vi "Dashboard Main.vi"() -> ()   [LabVIEW 2015]
uses:
  <vilib>/Utility/miscctls.llb/LVRowAndColumnTypeDef.ctl
  <vilib>/event_ctls.llb/eventvkey.ctl
  <vilib>/Rock Robotics/Network Tables/NT Read Boolean.vi
  <vilib>/Rock Robotics/WPI/Dashboard/WPI_DashboardLogging Global.vi
  <vilib>/Rock Robotics/Network Tables/NT Read Numeric Array.vi
  <vilib>/Utility/config.llb/Write Key (String).vi
  <vilib>/Utility/config.llb/Write Key (I32).vi
  <vilib>/Utility/config.llb/NI_LVConfig.lvlib
  <vilib>/vision/NI_Vision_Development_Module.lvlib
panel:
  out "Camera Image 2":T1(plugin-control)
  in  "Vision 2":u16(ring) items=["Camera Off", "USB Camera SW", "USB Camera HW", "IP Camera"]
  in  "Rec Mode":enum32{"Stop", "Record", "Playback"}(radio)
  in  "Vision":u16(ring) items=["Camera Off", "USB Camera SW", "USB Camera HW", "IP Camera"]
  in  "Dashboard Tab":T2(tab)
  out "Camera Reversed":bool
  out "dist":dbl
  in  "Select Auto":string(combo)
  out "NT Connection":bool
  in  "Camera Settings":T3={"Frame Rate"=30, "Compression"=30, "Size"=1} {"Frame Rate" scale=1.0..30.0; "Size" items=["640x480", "320x240", "160x120"]}
  out "MotorChart R":cluster{"Numeric":dbl, "Numeric":dbl}(graph)
  out "MotorChart L":T4(graph)
  out "MotorSliders R":cluster{"MotorSlide1":dbl, "MotorSlide2":dbl} {"MotorSlide2" scale=-1.0..1.0 scale format="%#_2e"; "MotorSlide1" scale=-1.0..1.0 scale format="%#_2e"}
  out "MotorSliders L":T5 {"MotorSlide4 2" scale=0.0..14.0 scale format="%#_2e"; "MotorSlide2" scale=-1.0..1.0 scale format="%#_2e"; "MotorSlide1" scale=-1.0..1.0 scale format="%#_2e"}
  out "Gyro":dbl(knob) scale=0.0..360.0
  out "JS1 Z":dbl(slide) scale=-1.0..1.0 scale format="%#_2e"
  out "JS1 Graph":cluster{"X":dbl, "Y":dbl}[](graph)
  out "JS1 Buttons":T6
  out "JS2 Z":dbl(slide) scale=-1.0..1.0 scale format="%#_2e"
  out "JS2 Graph":cluster{"X":dbl, "Y":dbl}[](graph)
  out "JS2 Buttons":T6
  out "Mode":T7(ring)=enum."Auto Disabled"
  in  "DB Camera Config":bool
  out "fps":dbl format="%#.1g"
  out "Mbps":dbl format="%#.1g"
  out "Mbps LED":bool
  in  "Camera Settings 2":T3={"Frame Rate"=30, "Compression"=30, "Size"=1} {"Frame Rate" scale=1.0..30.0; "Size" items=["640x480", "320x240", "160x120"]}
  out "Mbps 2":dbl format="%#.1g"
  out "fps 2":dbl format="%#.1g"
  out "Background":bool
  in  "DB/String 9":string
  in  "DB/String 8":string
  in  "DB/String 7":string
  in  "DB/String 6":string
  in  "DB/String 5":string
  in  "DB/String 4":string
  in  "DB/String 3":string
  in  "DB/String 2":string
  in  "DB/String 1":string
  in  "DB/String 0":string
  in  "DB/Slider 0":dbl(slide) scale=0.0..5.0
  in  "DB/Slider 1":dbl(slide) scale=0.0..5.0
  in  "DB/Slider 2":dbl(slide) scale=0.0..5.0
  in  "DB/Slider 3":dbl(slide) scale=0.0..5.0
  out "DB/LED 3":bool
  out "DB/LED 2":bool
  out "DB/LED 1":bool
  out "DB/LED 0":bool
  in  "DB/Button 3":bool
  in  "DB/Button 2":bool
  in  "DB/Button 1":bool
  in  "DB/Button 0":bool caption="New Name"
  in  "Test Slider":dbl(slide) scale=0.0..100.0 scale format="%#_3g"
  in  "On/Off":bool caption="Solenoid"
  in  "Test Name":u16(ring) items=["Select the test to run..."]
  in  "Test Tree":string(tree)
  in  "Motor":cluster{"Value":dbl, "Enable":bool} {"Value" scale=-1.0..1.0 scale format="%#_3g"}
  out "Progress":T8 {"Test Progress" scale=0.0..100.0}
  in  "Rev/Fwd":cluster{"Forward":bool, "Reverse":bool}
  in  "Test Ring":u16(ring) items=["Monochrome", "Color"]
  out "Cmd Status":string
  in  "Execute Command":bool
  in  "Command Params":string[][](table)
  in  "Command Selection":i32(listbox)
  in  "CheckList":i32(listbox)
  out "Tree":string(tree)
  in  "TCP":refnum<k5>
  out "Camera IP":string
  out "Image Message":string="Timeout in Camera Communications"
  out "Camera Image":T1(plugin-control)
  # "Left"
  # "Front"
  # "Right"
  # "Battery"
  # "This tab is a great place for autonomous settings and robot-specific values.\nPlace controls and indicators inside this tab and match name to\nDashboard Variables on robot. You can also delete this comment."
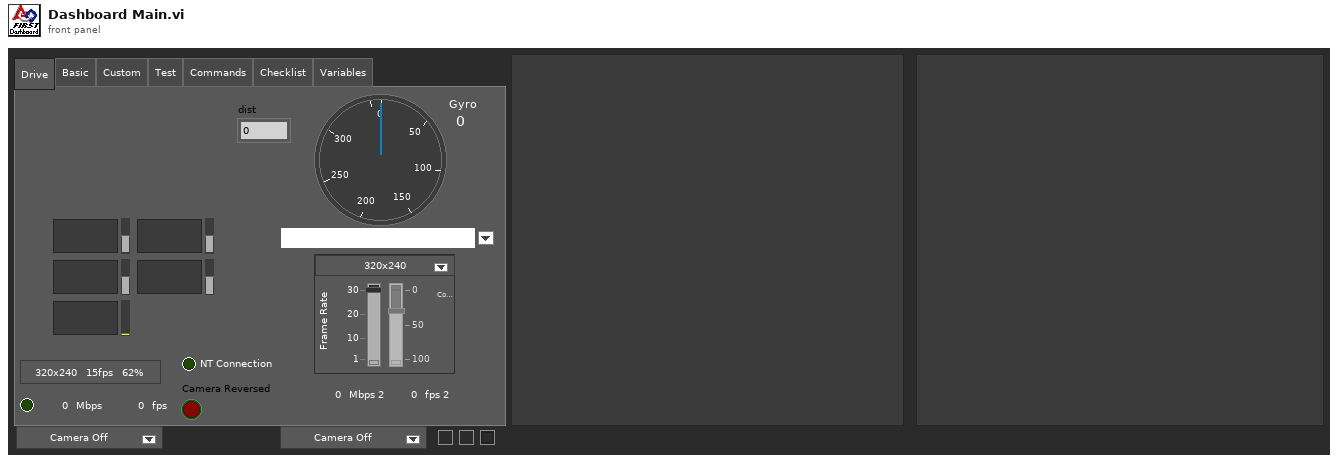
[diagram p1: front panel]
types:
  T1 = typedef "IMAQ Image.ctl" = refnum<image>
  T2 = enum32{"Drive", "Basic", "Custom", "Test", "Commands", "Checklist", "Variables"}
  T3 = cluster{"Frame Rate":i32, "Compression":i32, "Size":u16}
  T4 = cluster{"Numeric":dbl, "Numeric":dbl, "Battery V":dbl}
  T5 = cluster{"MotorSlide1":dbl, "MotorSlide2":dbl, "MotorSlide4 2":dbl}
  T6 = cluster{bool, bool, bool, bool, bool, bool, bool, bool, bool, bool, bool, bool}
  T7 = enum8{"Tele-Op Disabled", "Tele-Op Enabled", "Auto Disabled", "Auto Enabled", "Test Disabled", "Test Enabled", "Disconnected", "No Code", "E-Stop"}
  T8 = cluster{"Test Progress":u8, "Test Progress Text":string}
  T9 = cluster{"IDs":cluster{"RPC field ID":u16, "Unique ID":u16}, "String":string}
  T10 = enum32{"Drive", "Basic", "Custom", "Test", "Checklist", "Variables"}
  T11 = typedef "Image Type" = u32
  T12 = cluster{"Camera Image":refnum<vi>, "Dashboard Tab":refnum<vi>, "Background":refnum<vi>, "Vision":refnum<vi>, "Rec Mode":refnum<vi>, "Test Slider":refnum<vi>, "On/Off ":refnum<vi>, "Test Ring":refnum<vi>, "Rev/Fwd":refnum<vi>, "Test Name":refnum<vi>, "Motor":refnum<vi>, "Progress":refnum<vi>, "CheckList":refnum<vi>, "Tree":refnum<vi>, "Test Tree":refnum<vi>, "Command Params":refnum<vi>, "Command Selection":refnum<vi>, "Execute Command":refnum<vi>, "Cmd Status":refnum<vi>}
  T13 = cluster{"Error Strings":string, "Disable Counts":cluster{u16, u16}, "Rail Faults":cluster{u16, u16, u16}, "Robot IP":string, "DB Mode":u8, "Event Info":cluster{"Name":string, "Type":u8, "Number":u16, "Replay":u8}, "Camera Addr":string}
  T14 = cluster{"Storage":cluster{"Disk Free":u64, "RAM Block":u32, "RAM free":u32}, "CPU Utilization":cluster{"CPU % ISR":sgl, "CPU % Time Crit":sgl, "CPU % Timed Str":sgl, "CPU % High":sgl, "CPU % Above":sgl, "CPU % Normal":sgl, "CPU % Low":sgl}, "CAN":cluster{"% Bus Utilization":sgl, "Bus Off Cnt":u32, "TX_FIFO Full Cnt":u32, "Receive Error Cnt":u8, "Transmit Error Cnt":u8}, "HID":cluster{"HID Outputs":u32, "Rumble Low":u16, "Rumble High":u16}[]}
  T15 = cluster{"Status bits":cluster{"Test Mode":bool, "Autonomous":bool, "Enabled":bool, "Code Start":bool, "Brownout":bool, "Reserved 2":bool, "Reserved 3":bool, "E-Stop":bool}, "Code Trace":cluster{"Disabled":bool, "TeleOp":bool, "Auto":bool, "Test":bool}, "Controller Type":enum16{"unknown", "cRIO", "roboRio"}, "Code?":enum16{"unknown", "noCode", "code"}, "Battery V":dbl}
  T16 = cluster{"Control Bits":cluster{"TestMode":bool, "Autonomous":bool, "Enabled":bool, "FMS Present":bool, bool, bool, bool, "E-Stop":bool}, "Team Station ":u8, "Countdown":sgl, "Joystick Values":cluster{"Axes":dbl[], "Buttons":bool[], "POVs":i16[]}[]}
  T17 = cluster{"Axes":dbl[], "Buttons":bool[], "POVs":i16[]}[]
  T18 = cluster{"Axes":dbl[], "Buttons":bool[], "POVs":i16[]}
  T19 = cluster{"Buttons[0]":bool, "Buttons[1]":bool, "Buttons[2]":bool, "Buttons[3]":bool, "Buttons[4]":bool, "Buttons[5]":bool, "Buttons[6]":bool, "Buttons[7]":bool, "Buttons[8]":bool, "Buttons[9]":bool, "Buttons[10]":bool, "Buttons[11]":bool}
  T20 = typedef "NI_LVConfig.lvlib/Config Data RefNum.ctl" = refnum<k1>
  T21 = cluster{"Operation":enum16{"Update", "Clear"}, "Color Box":u32}[]
  T22 = typedef "eventvkey.ctl" = enum16{"ASCII", "Enter", "Return", "Shift", "Ctrl", "Alt", "Cmd", "Opt", "Caps", "NumLock", "Clear", "Break", "Up", "Down", "Left", "Right", "Insert", "Delete", "Home", "End", "PageUp", "PageDown", "Escape", "Help", "Pause", "ScrollLock", "F1", "F2", "F3", "F4", "F5", "F6", "F7", "F8", "F9", "F10", "F11", "F12", "F13", "F14", "F15", "F16", "F17", "F18", "F19", "F20", "F21", "F22", "F23", "F24", "Play", "VolumeUp", "VolumeDown", "Mute", "Two Byte Char"}
  T23 = cluster{"Image Size":bool, "Image Type":bool, "Pixel Value":bool, "ROI Information":bool, "Zoom Factor":bool}
  T24 = enum8{"Enabled", "Disabled", "Disabled and Grayed Out"}
  T25 = cluster{"Operation":enum16{"Update", "Clear"}, "Color Box":u32}
  T26 = typedef "LVRowAndColumnTypeDef.ctl" = cluster{"Row":i32, "Column":i32}
  T27 = cluster{"Shift":bool, "Ctrl":bool, "Alt":bool, "Cmd":bool, "Opt":bool}
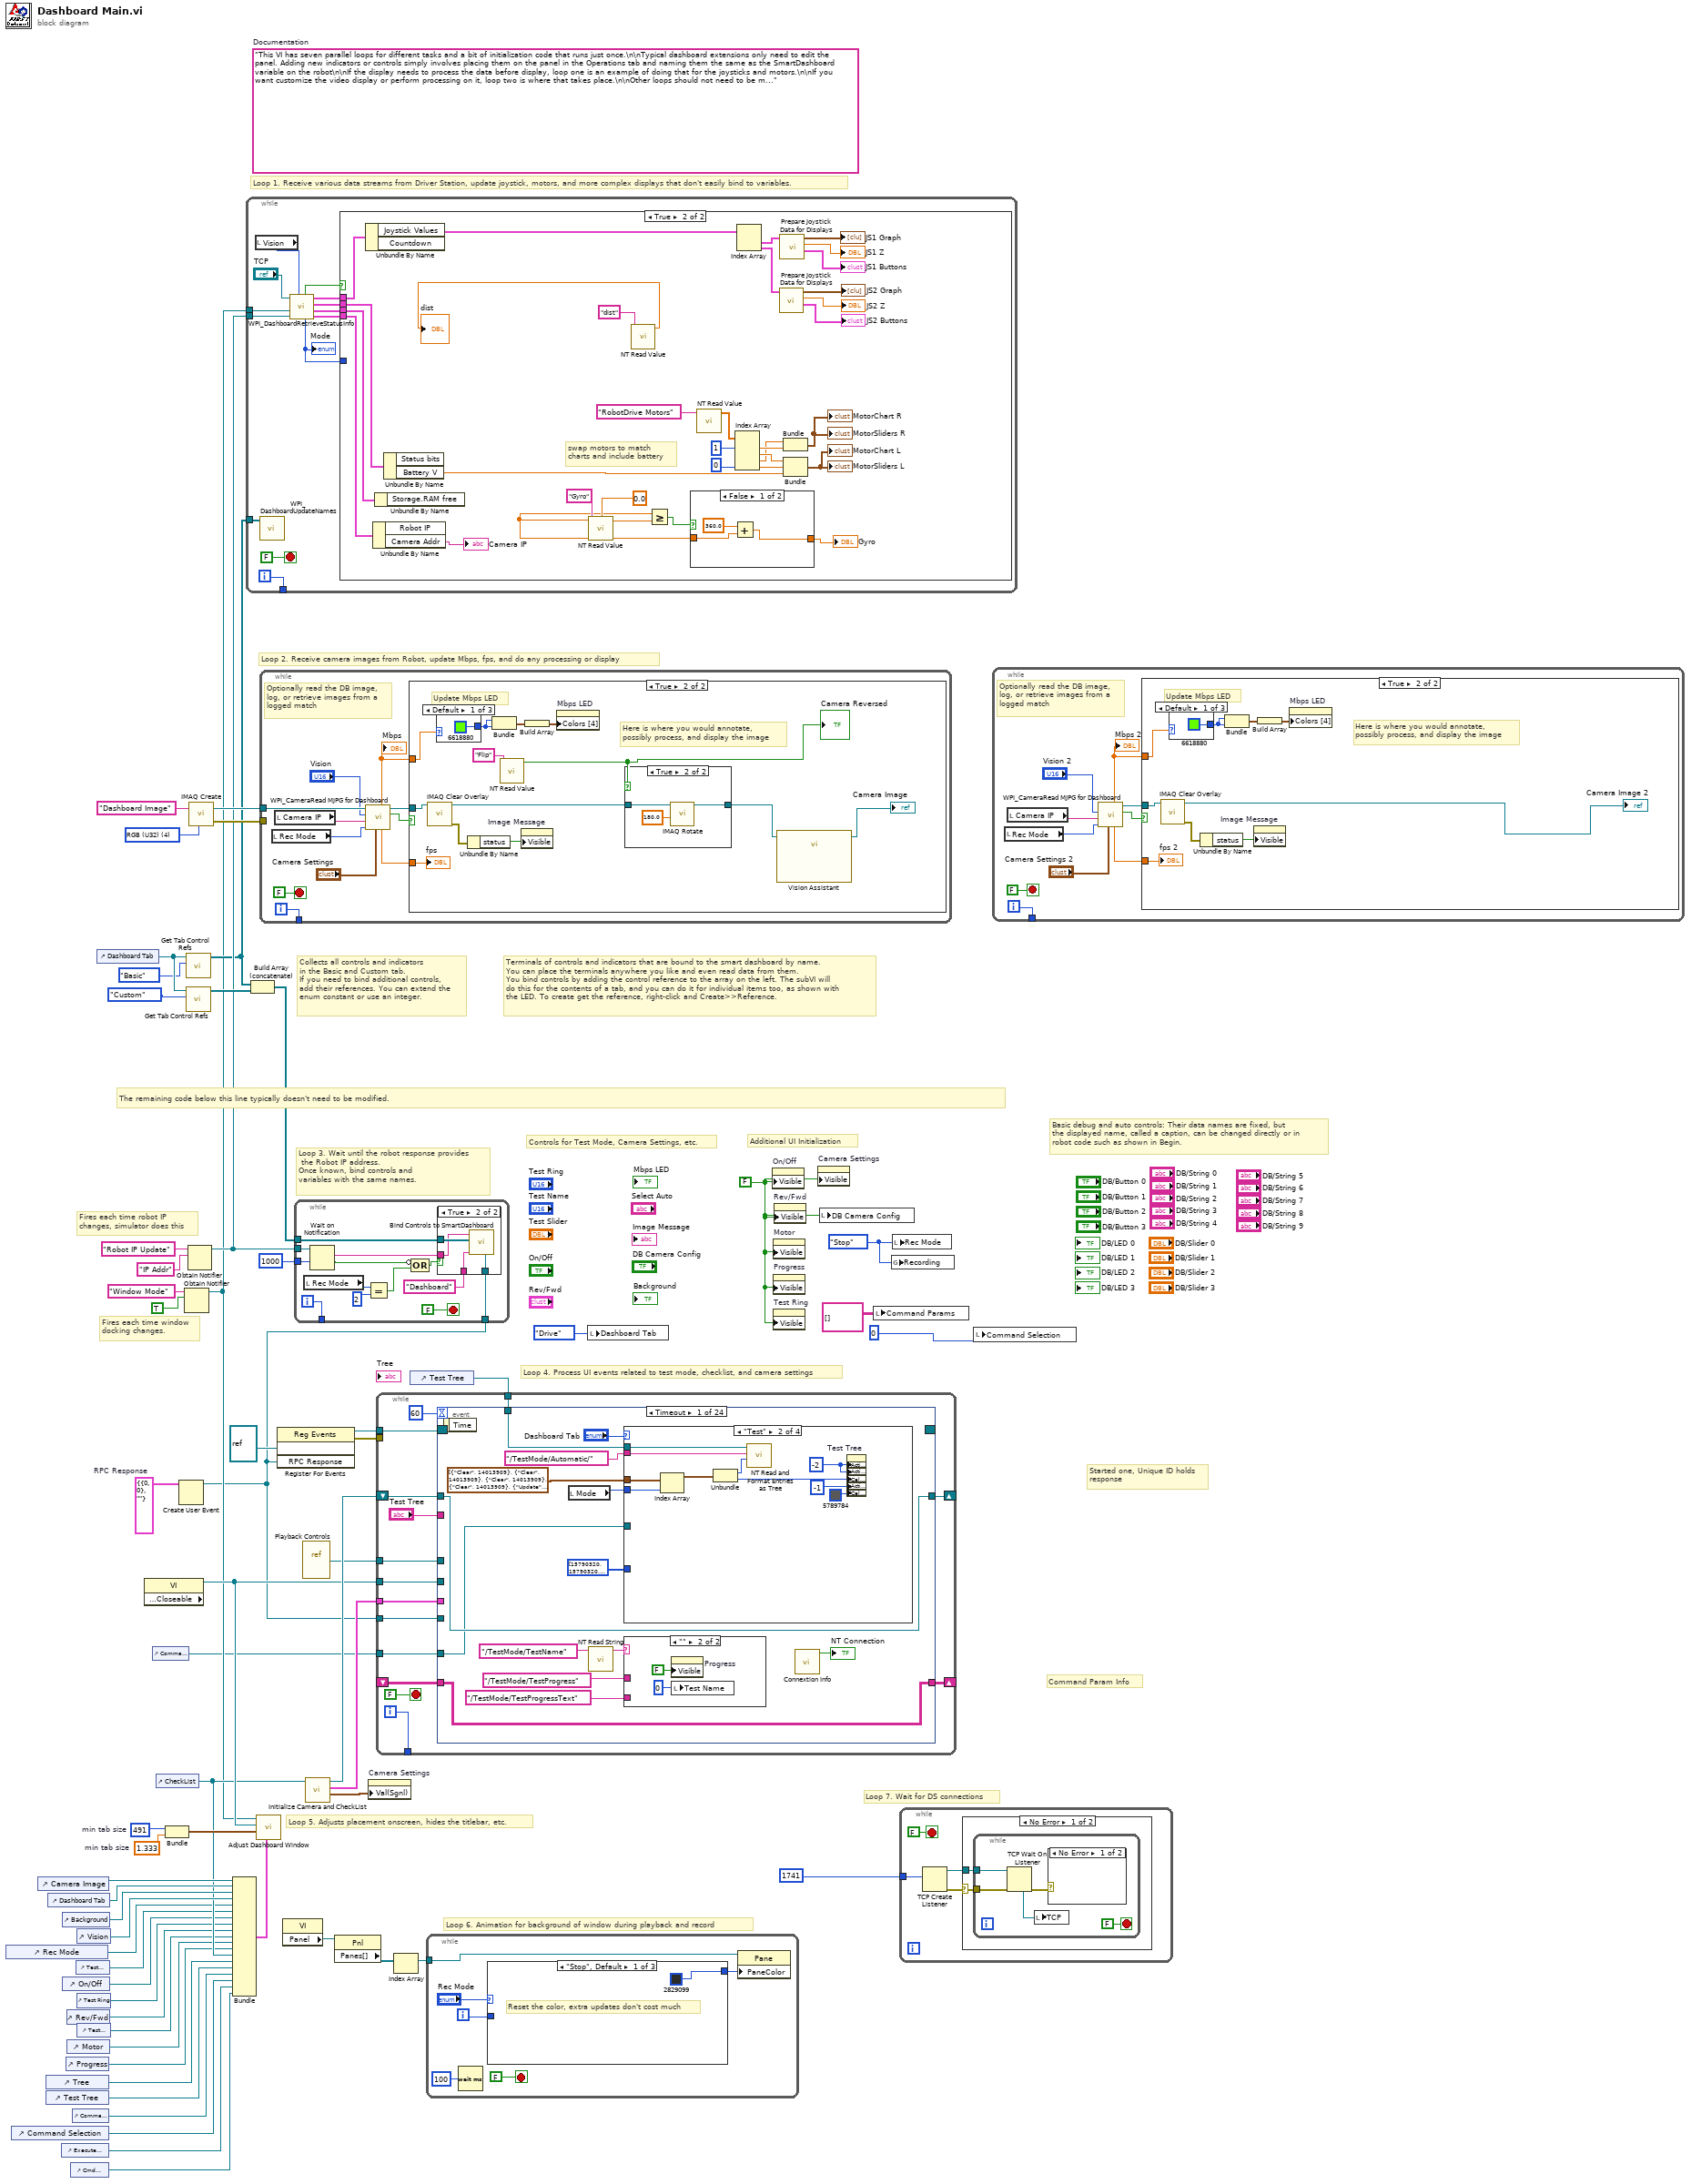
[diagram p0: block diagram]
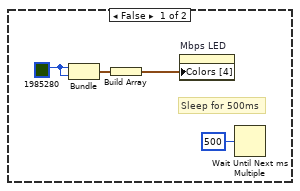
[diagram p2: hidden frame]
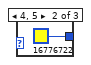
[diagram p3: hidden frame]
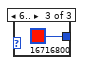
[diagram p4: hidden frame]
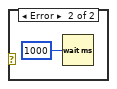
[diagram p5: hidden frame]
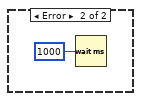
[diagram p6: hidden frame]
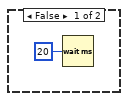
[diagram p7: hidden frame]
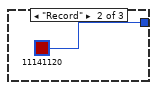
[diagram p9: hidden frame]
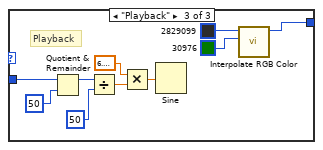
[diagram p10: hidden frame]
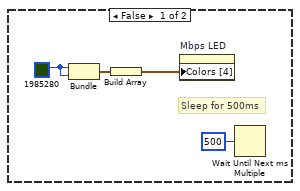
[diagram p12: hidden frame]
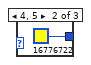
[diagram p14: hidden frame]
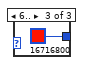
[diagram p15: hidden frame]
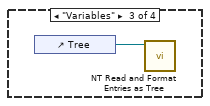
[diagram p17: hidden frame]
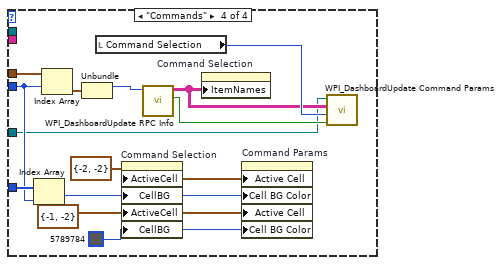
[diagram p18: hidden frame]
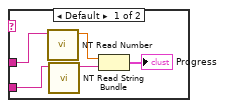
[diagram p19: hidden frame]
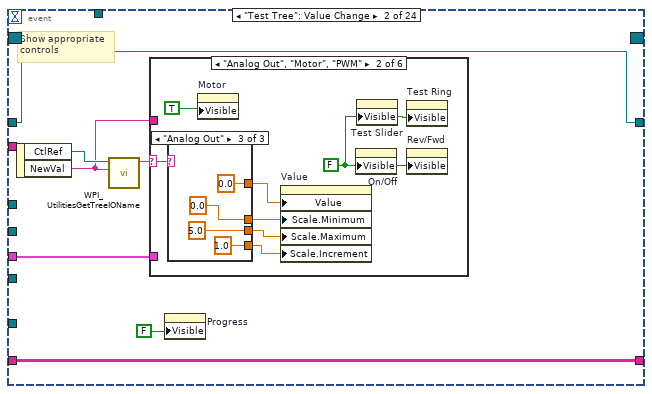
[diagram p20: hidden frame]
diagram:
  w7 = T9 {"IDs"={"RPC field ID"=0, "Unique ID"=0}, "String"=""}  # RPC Response
  w33 = 491  # min tab size
  w32 = 1.333  # min tab size
  w41 = enum32{"Stop", "Record", "Playback"}."Stop" ("Rec Mode")
  w15 = FALSE ("Visible")
  (unwired) "This VI has seven parallel loops for different tasks and a bit of initialization code that runs just once.\n\nTypical dashboard extensions only need to edit the panel. Adding new indicators or controls simply involves placing them on the panel in the Operations tab and naming them the same as the SmartDashboard variable on the robot\n\nIf the display needs to process the data before display, loop one is an example of doing that for the joysticks and motors.\n\nIf you want customize the video display or perform processing on it, loop two is where that takes place.\n\nOther loops should not need to be modified. They are pretty standard, and document the task they perform."  # Documentation
  w61 = T11 4 items=["Grayscale (U8)", "Grayscale (I16)", "Grayscale (SGL)", "Complex (CSG)", "RGB (U32)", "HSL (U32)", "RGB (U64)"] ("Image Type")
  # "Command Param Info"
  # "Started one, Unique ID holds\nresponse"
  # "Loop 7. Wait for DS connections"
  # "Basic debug and auto controls: Their data names are fixed, but\nthe displayed name, called a caption, can be changed directly or in\nrobot code such as shown in Begin."
  # "Controls for Test Mode, Camera Settings, etc."
  # "Additional UI Initialization"
  # "Loop 6. Animation for background of window during playback and record"
  # "Fires each time robot IP\nchanges, simulator does this"
  # "Fires each time window\ndocking changes."
  # "Collects all controls and indicators\nin the Basic and Custom tab.\nIf you need to bind additional controls,\nadd their references. You can extend the\nenum constant or use an integer."
  # "The remaining code below this line typically doesn't need to be modified."
  # "Loop 4. Process UI events related to test mode, checklist, and camera settings"
  # "Terminals of controls and indicators that are bound to the smart dashboard by name.\nYou can place the terminals anywhere you like and even read data from them.\nYou bind controls by adding the control reference to the array on the left. The subVI will\ndo this for the contents of a tab, and you can do it for individual items too, as shown with\nthe LED. To create get the reference, right-click and Create>>Reference."
  # "Loop 3. Wait until the robot response provides\n the Robot IP address.\nOnce known, bind controls and\nvariables with the same names."
  # "Loop 5. Adjusts placement onscreen, hides the titlebar, etc."
  # "Loop 1. Receive various data streams from Driver Station, update joystick, motors, and more complex displays that don't easily bind to variables."
  # "Loop 2. Receive camera images from Robot, update Mbps, fps, and do any processing or display"
  n1 = control-ref of="Rec Mode"() -> (w21:refnum<vi>)
  n2 = control-ref of="Command Selection"() -> (w6:refnum<vi>)
  n3 = control-ref of="Camera Image"() -> (w36:refnum<vi>)
  n4 = control-ref of="Tree"() -> (w25:refnum<vi>)
  n5 = control-ref of="Test Tree"() -> (w24:refnum<vi>)
  n6 = control-ref of="Dashboard Tab"() -> (w35:refnum<vi>)
  n7 = control-ref of="Execute Command"() -> (w8:refnum<vi>)
  n8 = control-ref of="Background"() -> (w30:refnum<vi>)
  n9 = control-ref of="On/Off"() -> (w19:refnum<vi>)
  n10 = control-ref of="Progress"() -> (w16:refnum<vi>)
  n11 = control-ref of="Rev/Fwd"() -> (w17:refnum<vi>)
  n12 = control-ref of="Motor"() -> (w22:refnum<vi>)
  n13 = control-ref of="Cmd Status"() -> (w2:refnum<vi>)
  n14 = control-ref of="Command Params"() -> (w9:refnum<vi>)
  n15 = control-ref of="Test Slider"() -> (w20:refnum<vi>)
  n16 = control-ref of="Vision"() -> (w34:refnum<vi>)
  n17 = control-ref of="Test Ring"() -> (w18:refnum<vi>)
  n18 = control-ref of="Test Name"() -> (w23:refnum<vi>)
  n19 = control-ref of="Dashboard Tab"() -> (w39:refnum<vi>)
  n20 = property class="VI" props=["Front Panel.Closeable"]() -> (reference out=w40:refnum<vi>)  [unwired: 2 in, 2 out]
  n21 = control-ref of="Command Params"() -> (w1:refnum<vi>)
  n22 = control-ref of="CheckList"() -> (w26:refnum<vi>)
  n23 = Bundle("min tab size"=w33, "min tab size"=w32) -> (w31:cluster{"min tab size":i32, "min tab size":dbl})  [unwired: 1 in]
  n24 = Create User Event(user event datatype=w7) -> (user event=w3:refnum<user-event>)  [unwired: 1 in, 1 out]
  n25 = Obtain Notifier(name (unnamed)="Window Mode", notification data type=TRUE) -> (notifier out=w12:refnum<notifier>)  [unwired: 2 in, 2 out]
  n26 = call <vilib>:"Get Tab Control Refs.vi"("Page Index"=T10."Basic" ("Dashboard Tab"), "TabControl in"=w39) -> ("ControlsOnPage"=w13:refnum<vi>[])  [unwired: 9 in]
  n27 = call <vilib>:"Get Tab Control Refs.vi"("Page Index"=T10."Custom" ("Dashboard Tab"), "TabControl in"=w39) -> ("ControlsOnPage"=w38:refnum<vi>[])  [unwired: 9 in]
  n28 = Obtain Notifier(name (unnamed)="Robot IP Update", notification data type="IP Addr" ("name (unnamed)")) -> (notifier out=w14:refnum<notifier>)  [unwired: 2 in, 2 out]
  n29 = call "IMAQ Create"("Image Name"="Dashboard Image", "Image Type"=w61) -> ("New Image"=w59:T1, "error out"=w58:errorcluster)  [unwired: 2 in, 1 out]
  n30 = Bundle("Camera Image"=w36, "Dashboard Tab"=w35, "Background"=w30, "Vision"=w34, "Rec Mode"=w21, "Test Slider"=w20, "On/Off"=w19, "Test Ring"=w18, "Rev/Fwd"=w17, "Test Name"=w23, "Motor"=w22, "Progress"=w16, "CheckList"=w26, "Tree"=w25, "Test Tree"=w24, "Command Params"=w9, "Command Selection"=w6, "Execute Command"=w8, "Cmd Status"=w2) -> (w27:T12)  [unwired: 1 in]
  n31 = while {
    tunnel: [w73] -> _
    tunnel: w14 -> [w67]
    tunnel: w13 -> [w66]
    tunnel: w12 -> [w62]
    i -> [w73]
    stop <- FALSE stop-if-true
    n32 = local read "Vision"() -> (w64:u16)
    n33 = call <vilib>:"WPI_DashboardUpdateNames.vi"("Controls on Tab"=w66) -> ()  [unwired: 11 in]
    n34 = call <vilib>:"WPI_DashboardRetrieveStatusInfo.vi"("Vision"=w64, "Binding Refnum"=w67, "Window Mode Notifier"=w62, "TCP Cnx"="TCP") -> ("Power and Errors"=w68:T13, "Robot Metrics"=w71:T14, "Status Info"=w72:T15, "Control Info"=w69:T16, "Robot Mode"=w65:T7, "Process?"=w70:bool)  [unwired: 2 in]
    "Mode" <- w65
    n35 = case shown="True" w70 {
      tunnel: w72 -> [_ w107]
      tunnel: w71 -> [_ w106]
      tunnel: w69 -> [_ w105]
      tunnel: w68 -> [_ w104]
      tunnel: w65 -> [_ _]
      frame False {
        n36 = Wait (ms)(milliseconds to wait=u32 20) -> ()  [unwired: 1 out]
      }
      frame True {
        # "swap motors to match\ncharts and include battery"
        n37 = Unbundle By Name(w105) -> ("Joystick Values"=w94:T17)  [unwired: 1 out]
        n38 = Unbundle By Name(w104) -> ("Camera Addr"=→"Camera IP":string)  [unwired: 1 out]
        n39 = Unbundle By Name(w106) -> ()  [unwired: 1 out]
        n40 = Unbundle By Name(w107) -> ("Battery V"=w95:dbl)  [unwired: 1 out]
        n41 = call-poly <vilib>:"NT Read Value.vi"("Name"="Gyro") -> ("Numeric"=w79:dbl)  [unwired: 9 in, 1 out]
        n42 = call-poly <vilib>:"NT Read Value.vi"("Name"="dist") -> ("Numeric"=→"dist":dbl)  [unwired: 9 in, 1 out]
        n43 = Greater Or Equal?(x=w79, y=0.0) -> (x >= y?=w81:bool)
        n44 = case shown="False" w81 {
          tunnel: [w108 w111] -> w78
          tunnel: w79 -> [w109 w111]
          frame False {
            n45 = Add(x=360.0, y=w109) -> (x+y=w108:dbl)
          }
          frame True {
          }
        }
        "Gyro" <- w78
        n46 = call-poly <vilib>:"NT Read Value.vi"("Name"="RobotDrive Motors") -> ("Numeric Array"=w83:dbl[])  [unwired: 9 in, 1 out]
        n47 = Index Array(array=w83, index #1=1, index #4=0) -> (element #1=w99:dbl, element #2=w100:dbl, element #3=w98:dbl, element #4=w103:dbl)  [unwired: 2 in]
        n48 = Index Array(array=w94) -> (element #1=w93:T18, element #2=w88:T18)  [unwired: 2 in]
        n49 = call "Prepare Joystick Data for Displays.vi"("Joystick Values"=w88) -> ("Buttons"=→"JS2 Buttons":T19, "Z Axis"=→"JS2 Z":dbl, "Cartesian Data"=→"JS2 Graph":cluster{"X axis":dbl, "X axis":dbl}[])  [unwired: 8 in]
        n50 = call "Prepare Joystick Data for Displays.vi"("Joystick Values"=w93) -> ("Buttons"=→"JS1 Buttons":T19, "Z Axis"=→"JS1 Z":dbl, "Cartesian Data"=→"JS1 Graph":cluster{"X axis":dbl, "X axis":dbl}[])  [unwired: 8 in]
        n51 = Bundle("Numeric"=w98, "Numeric"=w99) -> (→"MotorChart R" →"MotorSliders R":cluster{"Numeric":dbl, "Numeric":dbl})  [unwired: 1 in]
        n52 = Bundle("Numeric"=w100, "Numeric"=w103, "Battery V"=w95) -> (→"MotorChart L" →"MotorSliders L":T4)  [unwired: 1 in]
      }
    }
  }
  n53 = Build Array (concatenate)(w13, w38) -> (w37:refnum<vi>[])
  n54 = call "Adjust Dashboard Window.vi"("Sizing Refnums"=w27, "Size Constraints"=w31, "VI"=w40, "WIn Mode"=w12) -> ()  [unwired: 8 in]
  n55 = while {
    tunnel: w59 -> [w120]
    tunnel: w58 -> [_]
    tunnel: [w121] -> _
    i -> [w121]
    stop <- FALSE stop-if-true
    # "Optionally read the DB image,\nlog, or retrieve images from a\nlogged match"
    n56 = local read "Rec Mode"() -> (w115:enum32{"Stop", "Record", "Playback"})
    n57 = local read "Camera IP"() -> (w113:string)
    n58 = call <vilib>:"WPI_CameraRead MJPG for Dashboard.vi"("Camera Settings"="Camera Settings", "Rec Mode"=w115, "Camera IP"=w113, "Camera Mode"="Vision", "Refnum in"=w120) -> ("Active"=w118:bool, "Refnum out"=w119:T1, "FPS"=w117:dbl, "Bandwidth (Mbps)"=w112:dbl)  [unwired: 3 in]
    "Mbps" <- w112
    n59 = case shown="True" w118 {
      tunnel: w119 -> [_ w134]
      tunnel: w112 -> [_ w133]
      tunnel: w117 -> [_ w132]
      frame False {
        w123 = u32 1985280 ("Color Box")
        # "Sleep for 500ms"
        n60 = Bundle("Color Box"=w123, "Color Box"=w123) -> (w125:cluster{"Color Box":u32, "Color Box":u32})  [unwired: 1 out]
        n61 = Build Array(w125) -> (w124:cluster{"Color Box":u32, "Color Box":u32}[])
        n62 = property on="Mbps LED" class="Bool (strict)"("Colors [4]"=w124) -> ()  [unwired: 2 in, 2 out]
        n63 = Wait Until Next ms Multiple(millisecond multiple=u32 500) -> ()  [unwired: 1 out]
      }
      frame True {
        # "Here is where you would annotate,\npossibly process, and display the image"
        # "Update Mbps LED"
        n64 = call "IMAQ Clear Overlay"("Image"=w134) -> ("error out"=w138:errorcluster, "Image Out"=w131:T1)  [unwired: 2 in, 7 out]
        n65 = case shown="Default" w133 {
          tunnel: [u32 6618880 ("Color Box") u32 16776722 ("Color Box") u32 16716800 ("Color Box")] -> w135
          frame Default {
          }
          frame 4, 5 {
          }
          frame 6.. {
          }
        }
        n66 = Unbundle By Name(w138) -> ("status"=w139:bool)
        n67 = Bundle("Color Box"=w135, "Color Box"=w135) -> (w137:cluster{"Color Box":u32, "Color Box":u32})  [unwired: 1 out]
        n68 = call-poly <vilib>:"NT Read Value.vi"("Name"="Flip") -> ("Boolean"=w129:bool)  [unwired: 9 in, 1 out]
        "Camera Reversed" <- w129
        n69 = property on="Image Message" class="Str"("Visible"=w139) -> ()  [unwired: 2 in, 2 out]
        n70 = Build Array(w137) -> (w136:cluster{"Color Box":u32, "Color Box":u32}[])
        n71 = property on="Mbps LED" class="Bool (strict)"("Colors [4]"=w136) -> ()  [unwired: 2 in, 2 out]
        n72 = case shown="True" w129 {
          tunnel: w131 -> [w140 w143]
          tunnel: [w140 w142] -> w128
          frame False {
          }
          frame True {
            n73 = call "IMAQ Rotate"("Angle (degrees)"=sgl 180.0, "Image Src"=w143) -> ("Image Dst Out"=w142:T1)  [unwired: 8 in, 1 out]
          }
        }
        n74 = call "Vision Assistant"("Image In"=w128) -> ("Image Out"=→"Camera Image":T1)  [unwired: 25 in, 1 out]
        "fps" <- w132
      }
    }
  }
  n75 = register-events(refnum<vi> refnum, w3) -> (reference out=w45:refnum<event-registration>, error out=w44:errorcluster)  [unwired: 2 in]
  n76 = property class="VI"() -> ("Panel"=w48:refnum<vi>)  [unwired: 2 in, 2 out]
  n77 = while {
    tunnel: w37 -> [w159]
    tunnel: w14 -> [w157]
    tunnel: [w155] -> _
    tunnel: u32 1000 ("milliseconds to wait") -> [w154]
    tunnel: w3 -> [w147]
    i -> [w155]
    stop <- FALSE stop-if-true
    n78 = local read "Rec Mode"() -> (w150:enum32{"Stop", "Record", "Playback"})
    n79 = Wait on Notification(notifier=w157, timeout in ms (-1)=w154) -> (notification=w156:string, timed out?=w152:bool)  [unwired: 2 in, 2 out]
    n80 = Equal?(x=w150, y=u16 2 ("Rec Mode")) -> (x = y?=w151:bool)
    n81 = Compound Arithmetic op=OR(invert w152, w151) -> (w153:bool)
    n82 = case shown="True" w153 {
      tunnel: w159 -> [_ w163]
      tunnel: w156 -> [_ w162]
      tunnel: "Dashboard" -> [_ w161]
      tunnel: w147 -> [_ w160]
      frame False {
      }
      frame True {
        n83 = call <vilib>:"Bind Controls to SmartDashboard.vi"("RPC ref"=w160, "Client Name"=w161, "Bound Control Refs"=w163, "Server IP Address"=w162) -> ()  [unwired: 8 in]
      }
    }
  }
  n84 = vi-ref "Playback Controls.vi"() -> (w46:refnum<vi>)
  n85 = call "Initialize Camera and CheckList.vi"("ListBox in"=w26) -> ("Cluster"=w52:cluster{"value":i32, "value":i32, "index":i32}, "Array"=w53:cluster{string[]}[], "File Refnum"=w51:T20)  [unwired: 8 in]
  n86 = property class="Pnl"(reference=w48) -> ("Panes[]"=w49:refnum<vi>[])  [unwired: 1 in, 2 out]
  n87 = property on="Camera Settings" class="Clust (strict)"("Val(Sgnl)"=w52) -> ()  [unwired: 2 in, 2 out]
  n88 = Index Array(array=w49) -> (element=w47:refnum<vi>)  [unwired: 1 in]
  n89 = control-ref of="Test Tree"() -> (w50:refnum<vi>)
  n90 = while {
    tunnel: w53 -> [w175]
    shift-right: [w174] -> _
    shift-left: w51 -> [w173]
    tunnel: [w172] -> _
    tunnel: w50 -> [w171]
    tunnel: w46 -> [w170]
    tunnel: w45 -> [w169]
    tunnel: w44 -> [_]
    tunnel: w40 -> [w168]
    tunnel: w3 -> [w167]
    tunnel: w1 -> [w166]
    shift-right: [w165] -> _
    shift-left: _ -> [w164]
    i -> [w172]
    stop <- FALSE stop-if-true
    n91 = event shown="[0] Timeout" {
      selector: w169 -> [_ _ _ _ _ _ _ _ _ _ _ _ _ _ _ _ _ _ _ _ _ _ _ _]
      dyn-events: [_ _ _ _ _ _ _ _ _ _ _ _ _ _ _ _ _ _ w484 _ _ _ _ _] -> _
      timeout: u32 60 ("milliseconds to wait") -> [_ _ _ _ _ _ _ _ _ _ _ _ _ _ _ _ _ _ _ _ _ _ _ _]
      tunnel: w171 -> [w188 _ _ _ _ _ _ _ _ _ _ _ _ _ _ _ _ _ _ _ _ _ _ _]
      tunnel: "Test Tree" -> [_ _ _ _ _ _ _ _ _ _ _ _ _ w447 w456 w459 w464 w473 _ _ _ _ _ _]
      tunnel: w175 -> [_ w226 _ _ _ _ _ _ _ _ _ w409 w440 _ _ _ _ _ _ _ _ _ _ _]
      tunnel: [w185 w225 w329 w335 w345 w349 w355 w367 w375 w381 w394 w408 w433 w446 w454 w458 w463 w472 w486 w502 w504 w512 w523 w528] -> w174
      tunnel: w173 -> [w185 w225 w329 w335 w345 w349 w355 w367 w375 w381 w394 w407 w433 w446 w454 w458 w463 w472 w486 w502 w504 w512 w523 w528]
      tunnel: w170 -> [_ _ _ _ _ _ _ _ _ _ _ _ _ _ _ _ _ _ w487 _ w507 _ _ _]
      tunnel: w168 -> [_ _ _ _ _ _ _ _ _ _ _ _ _ _ _ _ _ _ w482 _ _ _ _ _]
      tunnel: w167 -> [_ _ _ _ _ _ _ _ _ _ _ _ _ _ _ _ _ _ w478 _ _ _ _ _]
      tunnel: w166 -> [w180 _ _ _ _ _ w353 _ _ _ _ _ _ _ _ _ _ _ _ _ _ _ _ _]
      tunnel: [w179 w224 w328 w334 w344 w350 w351 w361 w372 w380 w393 w406 w432 w445 w453 w457 w462 w471 w477 w500 w503 w508 w516 w529] -> w165
      tunnel: w164 -> [w179 w224 w328 w334 w344 w350 w351 _ _ w380 w393 w406 w432 w445 w453 w457 w462 w471 w477 w500 w503 w508 w516 w529]
      event Timeout {
        n92 = event-data() -> ()  [unwired: 1 in, 1 out]
        n93 = local read "Mode"() -> (w182:T7)
        n94 = call <vilib>:"NT Read String.vi"("Name"="/TestMode/TestName") -> ("String"=w191:string)  [unwired: 9 in, 1 out]
        n95 = case shown="\"Test\"" "Dashboard Tab" {
          tunnel: w188 -> [_ w202 _ _]
          tunnel: "/TestMode/Automatic/" ("Name Pattern") -> [_ w201 _ _]
          tunnel: T21 [{"Operation"=enum."Clear", "Color Box"=14013909}, {"Operation"=enum."Clear", "Color Box"=14013909}, {"Operation"=enum."Clear", "Color Box"=14013909}, {"Operation"=enum."Clear", "Color Box"=14013909}, {"Operation"=enum."Update", "Color Box"=14013909}, {"Operation"=enum."Update", "Color Box"=16777215}, {"Operation"=enum."Clear", "Color Box"=14013909}, {"Operation"=enum."Clear", "Color Box"=14013909}, {"Operation"=enum."Clear", "Color Box"=14013909}] -> [_ w194 _ w211]
          tunnel: w182 -> [_ w193 _ w210]
          tunnel: u32[] [15790320, 15790320, 15790320, 15790320, 16777215, 16777215, 15790320, 15790320, 15790320] -> [_ _ _ w216]
          tunnel: w180 -> [_ _ _ w204]
          frame "Custom", Default {
          }
          frame "Test" {
            w200 = -2 ("Active Item:Row Number")
            n96 = Index Array(array=w194, index=w193) -> (element=w195:T25)
            n97 = Unbundle(w195) -> ("Operation"=w196:enum16{"Update", "Clear"}, "Color Box"=w197:u32)
            n98 = call <vilib>:"NT Read and Format Entries as Tree.vi"("Operation"=w196, "Name Pattern"=w201, "Tree Refnum"=w202) -> ()  [unwired: 7 in, 2 out]
            n99 = property on="Test Tree" class="Tree (strict)"("Active Item Row Number"=w200, "ActiveColNum"=w200, "CellBG"=w197, "Active Item Row Number"=-1 ("Active Item:Row Number"), "CellBG"=u32 5789784 ("Color Box")) -> ()  [unwired: 2 in, 2 out]
          }
          frame "Variables" {
            n100 = control-ref of="Tree"() -> (w203:refnum<vi>)
            n101 = call <vilib>:"NT Read and Format Entries as Tree.vi"("Tree Refnum"=w203) -> ()  [unwired: 9 in, 2 out]
          }
          frame "Commands" {
            w212 = u32 5789784 ("Color Box")
            w213 = T26 {"Row"=-1, "Column"=-2} ("Active Cell:Active Cell")
            w215 = T26 {"Row"=-2, "Column"=-2} ("Active Cell:Active Cell")
            n102 = Index Array(array=w216, index=w210) -> (element=w214:u32)
            n103 = Index Array(array=w211, index=w210) -> (element=w209:T25)
            n104 = Unbundle(w209) -> ("Operation"=w208:enum16{"Update", "Clear"})  [unwired: 1 out]
            n105 = local read "Command Selection"() -> (w207:i32)
            n106 = property on="Command Selection" class="MCListbox (strict)"("ActiveCell"=w215, "CellBG"=w214, "ActiveCell"=w213, "CellBG"=w212) -> ()  [unwired: 2 in, 2 out]
            n107 = call <vilib>:"WPI_DashboardUpdate RPC Info.vi"("Operation"=w208) -> ("update"=w206:bool, "commands"=w205:string[][])  [unwired: 9 in]
            n108 = property on="Command Selection" class="MCListbox (strict)"("ItemNames"=w205) -> ()  [unwired: 2 in, 2 out]
            n109 = property on="Command Params" class="Tbl (strict)"("Active Cell"=w215, "Cell BG Color"=w214, "Active Cell"=w213, "Cell BG Color"=w212) -> ()  [unwired: 2 in, 2 out]
            n110 = call <vilib>:"WPI_DashboardUpdate Command Params.vi"("Update"=w206, "NewVal"=w207, "Commands"=w205, "Param Tbl"=w204) -> ()  [unwired: 7 in, 1 out]
          }
        }
        n111 = case shown="\"\"" w191 {
          tunnel: "/TestMode/TestProgress" ("Name") -> [w218 _]
          tunnel: "/TestMode/TestProgressText" ("Name") -> [w217 _]
          frame Default {
            n112 = call <vilib>:"NT Read Number.vi"("Name"=w218) -> ("Numeric"=w219:dbl)  [unwired: 9 in, 1 out]
            n113 = call <vilib>:"NT Read String.vi"("Name"=w217) -> ("String"=w220:string)  [unwired: 9 in, 1 out]
            n114 = Bundle("Numeric"=w219, "String"=w220) -> (→"Progress":cluster{"Numeric":dbl, "String":string})  [unwired: 1 in]
          }
          frame "" {
            n115 = property on="Progress" class="Clust (strict)"("Visible"=FALSE) -> ()  [unwired: 2 in, 2 out]
            n116 = local write "Test Name"(u16 0) -> ()
          }
        }
        n117 = call <vilib>:"Connextion Info.vi"() -> ("Connected"=→"NT Connection":bool)  [unwired: 10 in, 1 out]
      }
      event "Test Tree": Value Change {
        # "Show appropriate\ncontrols"
        n118 = event-data() -> ("CtlRef"=w229:refnum<vi>, "NewVal"=w227:string)  [unwired: 1 in]
        n119 = call <vilib>:"WPI_UtilitiesGetTreeIOName.vi"("NewVal"=w227, "TreeControl in"=w229) -> ("I/O Name"=w230:string)  [unwired: 9 in]
        n120 = case shown="\"Analog Out\", \"Motor\", \"PWM\"" w230 {
          selector: w230 -> [_ w237 _ w259 w268 _]
          tunnel: w227 -> [_ _ w256 w258 _ w275]
          tunnel: w226 -> [_ _ _ _ _ w274]
          frame Default {
            w232 = FALSE ("Visible")
            w231 = FALSE ("Visible")
            n121 = property on="Motor" class="Clust (strict)"("Visible"=w231) -> ()  [unwired: 2 in, 2 out]
            n122 = property on="Test Ring" class="Ring (strict)"("Visible"=w231) -> ()  [unwired: 2 in, 2 out]
            n123 = property on="Rev/Fwd" class="Clust (strict)"("Visible"=w232) -> ()  [unwired: 2 in, 2 out]
            n124 = property on="On/Off" class="Bool (strict)"("Visible"=w232) -> ()  [unwired: 2 in, 2 out]
            n125 = property on="Test Slider" class="Slide (strict)"("Visible"=w232) -> ()  [unwired: 2 in, 2 out]
          }
          frame "Analog Out", "Motor", "PWM" {
            w238 = FALSE ("Visible")
            n126 = case shown="\"Analog Out\"" w237 {
              tunnel: [1.0 ("Value") -1.0 ("Value") 0.0 ("Value")] -> w236
              tunnel: [255.0 ("Value") 1.0 ("Value") 5.0 ("Value")] -> w235
              tunnel: [128.0 ("Value") 0.0 ("Value") 0.0 ("Value")] -> w234
              tunnel: [64.0 ("Value") 0.5 ("Value") 1.0 ("Value")] -> w233
              frame "PWM" {
              }
              frame "Motor", Default {
              }
              frame "Analog Out" {
              }
            }
            n127 = property on="Motor" class="Clust (strict)"("Visible"=TRUE) -> ()  [unwired: 2 in, 2 out]
            n128 = property on="Value" class="Slide (strict)"("Value"=w234, "Scale.Minimum"=w236, "Scale.Maximum"=w235, "Scale.Increment"=w233) -> ()  [unwired: 2 in, 2 out]
            n129 = property on="On/Off" class="Bool (strict)"("Visible"=w238) -> ()  [unwired: 2 in, 2 out]
            n130 = property on="Test Slider" class="Slide (strict)"("Visible"=w238) -> ()  [unwired: 2 in, 2 out]
            n131 = property on="Test Ring" class="Ring (strict)"("Visible"=w238) -> ()  [unwired: 2 in, 2 out]
            n132 = property on="Rev/Fwd" class="Clust (strict)"("Visible"=w238) -> ()  [unwired: 2 in, 2 out]
          }
          frame "Servo" {
            w254 = FALSE ("Visible")
            n133 = call <vilib>:"NT Read Number.vi"("Name"=w256) -> ("Numeric"=w255:dbl)  [unwired: 9 in, 1 out]
            n134 = property on="Test Slider" class="Slide (strict)"("Visible"=TRUE, "Scale.Maximum"=170.0 ("Scale.Range:Maximum")) -> ()  [unwired: 2 in, 2 out]
            n135 = local write "Test Slider"(w255) -> ()
            n136 = property on="Motor" class="Clust (strict)"("Visible"=w254) -> ()  [unwired: 2 in, 2 out]
            n137 = property on="Rev/Fwd" class="Clust (strict)"("Visible"=w254) -> ()  [unwired: 2 in, 2 out]
            n138 = property on="On/Off" class="Bool (strict)"("Visible"=w254) -> ()  [unwired: 2 in, 2 out]
            n139 = property on="Test Ring" class="Ring (strict)"("Visible"=w254) -> ()  [unwired: 2 in, 2 out]
          }
          frame "Relay", "Solenoid" {
            w257 = FALSE ("Visible")
            n140 = property on="Motor" class="Clust (strict)"("Visible"=w257) -> ()  [unwired: 2 in, 2 out]
            n141 = property on="Test Slider" class="Slide (strict)"("Visible"=w257) -> ()  [unwired: 2 in, 2 out]
            n142 = Search and Replace String(input string=w258, search string="/Value  **", replace string="/Direction") -> (result string=w264:string)  [unwired: 5 in, 3 out]
            n143 = property on="Test Ring" class="Ring (strict)"("Visible"=w257) -> ()  [unwired: 2 in, 2 out]
            n144 = call <vilib>:"NT Read String.vi"("Name"=w264) -> ("String"=w262:string)  [unwired: 9 in, 1 out]
            n145 = Equal?(x="Both directions", y=w262) -> (x = y?=w260:bool)
            n146 = Not(x=w260) -> (.not. x?=w261:bool)
            n147 = property on="Rev/Fwd" class="Clust (strict)"("Visible"=w260) -> ()  [unwired: 2 in, 2 out]
            n148 = property on="On/Off" class="Bool (strict)"("Visible"=w261, "Caption.Text"=w259) -> ()  [unwired: 2 in, 2 out]
          }
          frame "Compressor", "Digital Out" {
            w267 = FALSE ("Visible")
            # "Get direction and finish"
            n149 = property on="Motor" class="Clust (strict)"("Visible"=w267) -> ()  [unwired: 2 in, 2 out]
            n150 = property on="Test Slider" class="Slide (strict)"("Visible"=w267) -> ()  [unwired: 2 in, 2 out]
            n151 = property on="Test Ring" class="Ring (strict)"("Visible"=w267) -> ()  [unwired: 2 in, 2 out]
            n152 = property on="On/Off" class="Bool (strict)"("Visible"=TRUE, "Caption.Text"=w268) -> ()  [unwired: 2 in, 2 out]
            n153 = property on="Rev/Fwd" class="Clust (strict)"("Visible"=FALSE) -> ()  [unwired: 2 in, 2 out]
          }
          frame "Camera" {
            n154 = call <vilib>:"Get Last Path Segment.vi"("String in"=w275) -> ("String out"=w276:string)  [unwired: 10 in]
            n155 = property on="On/Off" class="Bool (strict)"("Visible"=FALSE) -> ()  [unwired: 2 in, 2 out]
            n156 = property on="Motor" class="Clust (strict)"("Visible"=FALSE) -> ()  [unwired: 2 in, 2 out]
            n157 = property on="Rev/Fwd" class="Clust (strict)"("Visible"=FALSE) -> ()  [unwired: 2 in, 2 out]
            n158 = case shown="\"White Balance  **\"" w276 {
              tunnel: w275 -> [w282 w291 w300 w309 w318 _ w324]
              tunnel: w274 -> [w280 w288 w297 w306 w315 _ _]
              frame "Size  **" {
                n159 = Index Array(array=w280) -> (element=w279:cluster{string[]})  [unwired: 1 in]
                n160 = call <vilib>:"NT Read String.vi"("Name"=w282) -> ("String"=w281:string)  [unwired: 9 in, 1 out]
                n161 = Unbundle(w279) -> (w277:string[])
                n162 = Match First String(2:w277, 3:w281) -> (0:w278:i32)  [unwired: 1 out]
                n163 = property on="Test Ring" class="Ring (strict)"("Value"=w278, "Strings []"=w277) -> ()  [unwired: 2 in, 2 out]
                n164 = property on="Test Ring" class="Ring (strict)"("Visible"=TRUE) -> ()  [unwired: 2 in, 2 out]
                n165 = property on="Test Slider" class="Slide (strict)"("Visible"=FALSE) -> ()  [unwired: 2 in, 2 out]
              }
              frame "White Balance  **" {
                n166 = Index Array(array=w288, index=1) -> (element=w289:cluster{string[]})
                n167 = call <vilib>:"NT Read String.vi"("Name"=w291) -> ("String"=w290:string)  [unwired: 9 in, 1 out]
                n168 = Unbundle(w289) -> (w286:string[])
                n169 = Match First String(2:w286, 3:w290) -> (0:w285:i32)  [unwired: 1 out]
                n170 = property on="Test Ring" class="Ring (strict)"("Value"=w285, "Strings []"=w286) -> ()  [unwired: 2 in, 2 out]
                n171 = property on="Test Ring" class="Ring (strict)"("Visible"=TRUE) -> ()  [unwired: 2 in, 2 out]
                n172 = property on="Test Slider" class="Slide (strict)"("Visible"=FALSE) -> ()  [unwired: 2 in, 2 out]
              }
              frame "Exposure  **" {
                n173 = Index Array(array=w297, index=2) -> (element=w298:cluster{string[]})
                n174 = call <vilib>:"NT Read String.vi"("Name"=w300) -> ("String"=w299:string)  [unwired: 9 in, 1 out]
                n175 = Unbundle(w298) -> (w294:string[])
                n176 = Match First String(2:w294, 3:w299) -> (0:w295:i32)  [unwired: 1 out]
                n177 = property on="Test Ring" class="Ring (strict)"("Value"=w295, "Strings []"=w294) -> ()  [unwired: 2 in, 2 out]
                n178 = property on="Test Ring" class="Ring (strict)"("Visible"=TRUE) -> ()  [unwired: 2 in, 2 out]
                n179 = property on="Test Slider" class="Slide (strict)"("Visible"=FALSE) -> ()  [unwired: 2 in, 2 out]
              }
              frame "Exposure Priority  **" {
                n180 = Index Array(array=w306, index=3) -> (element=w307:cluster{string[]})
                n181 = call <vilib>:"NT Read String.vi"("Name"=w309) -> ("String"=w308:string)  [unwired: 9 in, 1 out]
                n182 = Unbundle(w307) -> (w303:string[])
                n183 = Match First String(2:w303, 3:w308) -> (0:w304:i32)  [unwired: 1 out]
                n184 = property on="Test Ring" class="Ring (strict)"("Value"=w304, "Strings []"=w303) -> ()  [unwired: 2 in, 2 out]
                n185 = property on="Test Ring" class="Ring (strict)"("Visible"=TRUE) -> ()  [unwired: 2 in, 2 out]
                n186 = property on="Test Slider" class="Slide (strict)"("Visible"=FALSE) -> ()  [unwired: 2 in, 2 out]
              }
              frame "Color Enable  **" {
                n187 = Index Array(array=w315, index=4) -> (element=w316:cluster{string[]})
                n188 = call <vilib>:"NT Read String.vi"("Name"=w318) -> ("String"=w317:string)  [unwired: 9 in, 1 out]
                n189 = Unbundle(w316) -> (w312:string[])
                n190 = Match First String(2:w312, 3:w317) -> (0:w313:i32)  [unwired: 1 out]
                n191 = property on="Test Ring" class="Ring (strict)"("Value"=w313, "Strings []"=w312) -> ()  [unwired: 2 in, 2 out]
                n192 = property on="Test Ring" class="Ring (strict)"("Visible"=TRUE) -> ()  [unwired: 2 in, 2 out]
                n193 = property on="Test Slider" class="Slide (strict)"("Visible"=FALSE) -> ()  [unwired: 2 in, 2 out]
              }
              frame Default {
                n194 = property on="Test Ring" class="Ring (strict)"("Visible"=FALSE) -> ()  [unwired: 2 in, 2 out]
                n195 = property on="Test Slider" class="Slide (strict)"("Visible"=FALSE) -> ()  [unwired: 2 in, 2 out]
              }
              frame "Brightness  **", "Color Level  **", "Compression  **", "FPS  **", "Sharpness  **" {
                n196 = call <vilib>:"NT Read Number.vi"("Name"=w324) -> ("Numeric"=w323:dbl)  [unwired: 9 in, 1 out]
                n197 = local write "Test Slider"(w323) -> ()
                n198 = property on="Test Slider" class="Slide (strict)"("Visible"=TRUE, "Scale.Maximum"=100.0 ("Scale.Range:Maximum")) -> ()  [unwired: 2 in, 2 out]
                n199 = property on="Test Ring" class="Ring (strict)"("Visible"=FALSE) -> ()  [unwired: 2 in, 2 out]
              }
            }
          }
        }
        n200 = property on="Progress" class="Clust (strict)"("Visible"=FALSE) -> ()  [unwired: 2 in, 2 out]
      }
      event "Test Name": Mouse Enter {
        # "Populate the ring with the list of tests"
        n201 = event-data() -> ()  [unwired: 1 in, 1 out]
        n202 = call <vilib>:"NT Read String Array.vi"("Name"="/TestMode/TestList") -> ("String Array"=w333:string[])  [unwired: 9 in, 1 out]
        n203 = Build Array (concatenate)("Select the test to run...", w333) -> (w332:string[])
        n204 = property on="Test Name" class="Ring (strict)"("Strings []"=w332) -> ()  [unwired: 2 in, 2 out]
      }
      event "Test Name": Value Change {
        w336 = FALSE ("Visible")
        # "Tell the robot the test name to run"
        n205 = event-data() -> ("NewVal"=w340:u16)  [unwired: 1 in]
        n206 = property on="Test Name" class="Ring (strict)"() -> ("Strings []"=w341:string[])  [unwired: 2 in, 2 out]
        n207 = local write "Progress"(T8 {"Test Progress"=0, "Test Progress Text"=""} ("Progress")) -> ()
        n208 = Index Array(array=w341, index=w340) -> (element=w339:string)
        n209 = call <vilib>:"NT Write String.vi"("String"=w339, "Name"="/TestMode/TestName") -> ()  [unwired: 9 in, 1 out]
        n210 = property on="Progress" class="Clust (strict)"("Visible"=TRUE) -> ()  [unwired: 2 in, 2 out]
        n211 = property on="Motor" class="Clust (strict)"("Visible"=w336) -> ()  [unwired: 2 in, 2 out]
        n212 = property on="Test Slider" class="Slide (strict)"("Visible"=w336) -> ()  [unwired: 2 in, 2 out]
        n213 = property on="On/Off" class="Bool (strict)"("Visible"=w336) -> ()  [unwired: 2 in, 2 out]
        n214 = property on="Rev/Fwd" class="Clust (strict)"("Visible"=w336) -> ()  [unwired: 2 in, 2 out]
        n215 = property on="Test Ring" class="Ring (strict)"("Visible"=w336) -> ()  [unwired: 2 in, 2 out]
      }
      event "Select Auto": Mouse Enter {
        # "Populate the combo box with the list of autonomous options"
        n216 = event-data() -> ()  [unwired: 1 in, 1 out]
        n217 = call <vilib>:"NT Read String Array.vi"("Name"="Auto List") -> ("String Array"=w343:string[])  [unwired: 9 in, 1 out]
        n218 = property on="Select Auto" class="CmbBox"("Strings[]"=w343) -> ()  [unwired: 2 in, 2 out]
      }
      event "Select Auto": Value Change {
        # "User modified the Auto Selection. Write to NT variable so robot knows."
        n219 = event-data() -> ("NewVal"=w347:string)  [unwired: 1 in]
        n220 = call <vilib>:"NT Write String.vi"("String"=w347, "Name"="Auto Selector") -> ()  [unwired: 9 in, 1 out]
      }
      event "Command Selection": Value Change {
        # "Get the params and show in table"
        n221 = event-data() -> ("NewVal"=w354:i32)  [unwired: 1 in]
        n222 = property on="Command Selection" class="MCListbox (strict)"() -> ("ItemNames"=w352:string[][])  [unwired: 2 in, 2 out]
        n223 = call <vilib>:"WPI_DashboardUpdate Command Params.vi"("NewVal"=w354, "Commands"=w352, "Param Tbl"=w353) -> ()  [unwired: 8 in, 1 out]
      }
      event "Execute Command": Value Change {
        # "Started one, Unique ID holds\nresponse"
        n224 = event-data() -> ()  [unwired: 1 in, 1 out]
        n225 = property on="Command Selection" class="MCListbox (strict)"() -> ("ItemNames"=w366:string[][])  [unwired: 2 in, 2 out]
        n226 = Index Array(array=w366, index (row)="Command Selection", index (col)=0) -> (element=w364:string)
        n227 = call <vilib>:"Invoke Commands.vi"("Command Params"="Command Params", "Function Name"=w364) -> ("Params"=w360:u8, "Started"=w359:bool)  [unwired: 7 in, 1 out]
        n228 = Array Subset(array="Command Params", length (row)=w360) -> (w361:string[][])  [unwired: 3 in]
        n229 = Select(t="Executing" ("Cmd Status"), s=w359, f="" ("Cmd Status")) -> (s? t:f=→"Cmd Status":string)
      }
      event "Command Selection": Double Click {
        n230 = event-data() -> ("Row"=w376:i32)  [unwired: 1 in]
        n231 = property on="Command Selection" class="MCListbox (strict)"() -> ("ItemNames"=w379:string[][])  [unwired: 2 in, 2 out]
        n232 = local read "Command Params"() -> (w374:string[][])
        n233 = Index Array(array=w379, index (row)=w376, index (col)=0) -> (element=w377:string)
        n234 = call <vilib>:"Invoke Commands.vi"("Command Params"=w374, "Function Name"=w377) -> ("Params"=w373:u8, "Started"=w368:bool)  [unwired: 7 in, 1 out]
        n235 = Array Subset(array=w374, length (row)=w373) -> (w372:string[][])  [unwired: 3 in]
        n236 = Select(t="Executing" ("Cmd Status"), s=w368, f="" ("Cmd Status")) -> (s? t:f=w369:string)
        n237 = local write "Cmd Status"(w369) -> ()
      }
      event "CheckList": Double Click {
        # "Shift clears all"
        # "Update symbols on the listbox"
        n238 = event-data() -> ("PlatMods.Shift"=w382:bool, "Row"=w384:i32)  [unwired: 1 in]
        n239 = case shown="True" w382 {
          tunnel: w384 -> [w388 _]
          tunnel: 1 -> [w387 _]
          frame False {
            n240 = property on="CheckList" class="LstBox (strict)"() -> ("Item Symbols"=w386:i32[])  [unwired: 2 in, 2 out]
            n241 = Replace Array Subset(array=w386, new element=w387, index=w388) -> (w385:i32[])
            n242 = property on="CheckList" class="LstBox (strict)"("Item Symbols"=w385) -> ()  [unwired: 2 in, 2 out]
          }
          frame True {
            w389 = 0 ("Top Row")
            n243 = property on="CheckList" class="LstBox (strict)"() -> ("Number of Rows"=w391:u32)  [unwired: 2 in, 2 out]
            n244 = Initialize Array(0, w391) -> (w390:i32[])
            n245 = property on="CheckList" class="LstBox (strict)"("Top Row"=w389, "Value"=w389, "Item Symbols"=w390) -> ()  [unwired: 2 in, 2 out]
          }
        }
      }
      event "CheckList": Key Down {
        # "Update symbols on the listbox\nLeft and right keys check and uncheck"
        n246 = event-data() -> ("VKey"=w396:T22)  [unwired: 1 in]
        n247 = case shown="\"Left\", \"Right\"" w396 {
          selector: w396 -> [w401 _]
          tunnel: eventvkey."Left" ("VKey") -> [w399 _]
          frame "Left", "Right" {
            n248 = Equal?(x=w399, y=w401) -> (x = y?=w400:bool)
            n249 = Select(t=0, s=w400, f=1) -> (s? t:f=w402:i32)
            n250 = property on="CheckList" class="LstBox (strict)"() -> ("Item Symbols"=w405:i32[])  [unwired: 2 in, 2 out]
            n251 = Replace Array Subset(array=w405, new element=w402, index="CheckList") -> (w404:i32[])
            n252 = property on="CheckList" class="LstBox (strict)"("Item Symbols"=w404) -> ()  [unwired: 2 in, 2 out]
          }
          frame Default {
          }
        }
      }
      event "DB Camera Config": Value Change {
        # "Show or hide the cluster of controls, store in ini file"
        n253 = event-data() -> ("NewVal"=w410:bool)  [unwired: 1 in]
        n254 = case shown="False" w410 {
          tunnel: w409 -> [w419 _]
          tunnel: [w412 w430] -> w408
          tunnel: w407 -> [w411 w430]
          frame False {
            w426 = "Camera"
            w429 = FALSE ("Visible")
            n255 = local read "Camera Settings"() -> (w418:T3)
            n256 = Index Array(array=w419) -> (element=w422:cluster{string[]})  [unwired: 1 in]
            n257 = Unbundle(w418) -> ("Frame Rate"=w417:i32, "Compression"=w416:i32, "Size"=w420:u16)
            n258 = Unbundle(w422) -> (w421:string[])
            n259 = Index Array(array=w421, index=w420) -> (element=w415:string)
            n260 = call-poly <vilib>:"Write Key.vi"("section"=w426, "value"=w415, "key"="Size", "refnum"=w411) -> ("refnum out"=w428:T20)  [unwired: 2 in, 5 out]
            n261 = call-poly <vilib>:"Write Key.vi"("section"=w426, "value"=w417, "key"="FrameRate", "refnum"=w428) -> ("refnum out"=w427:T20)  [unwired: 1 in, 6 out]
            n262 = property on="Camera Settings" class="Clust (strict)"("Visible"=w429) -> ()  [unwired: 2 in, 2 out]
            n263 = local write "DB Camera Config"(w429) -> ()
            n264 = call-poly <vilib>:"Write Key.vi"("section"=w426, "value"=w416, "key"="Compression", "refnum"=w427) -> ("refnum out"=w413:T20)  [unwired: 1 in, 6 out]
            n265 = call <vilib>:"Close Config Data.vi"("refnum"=w413) -> ("file path"=w414:path)  [unwired: 2 in, 8 out]
            n266 = call <vilib>:"Open Config Data.vi"("configuration file path"=w414) -> ("refnum"=w412:T20)  [unwired: 8 in, 2 out]
          }
          frame True {
            n267 = property on="Camera Settings" class="Clust (strict)"("Visible"=TRUE) -> ()  [unwired: 2 in, 2 out]
          }
        }
      }
      event "Camera Settings": Value Change {
        # "Update summary string when any elements of DB camera change"
        n268 = event-data() -> ("NewVal"=w444:T3)  [unwired: 1 in]
        n269 = Index Array(array=w440) -> (element=w439:cluster{string[]})  [unwired: 1 in]
        n270 = Unbundle(w444) -> ("Frame Rate"=w435:i32, "Compression"=w434:i32, "Size"=w437:u16)
        n271 = Unbundle(w439) -> (w438:string[])
        n272 = Index Array(array=w438, index=w437) -> (element=w436:string)
        n273 = Format Into String(format string="%s   %dfps   %d%%", w436, w435, w434) -> (resulting string=w441:string)  [unwired: 2 in, 1 out]
        n274 = Build Array(w441) -> (w442:string[])
        n275 = property on="DB Camera Config" class="Bool (strict)"("Strings [4]"=w442) -> ()  [unwired: 2 in, 2 out]
      }
      event "Motor.Enable": Value Change {
        # "When the test mode otor enable helper is set, update that\ntree row item's value"
        n276 = event-data() -> ("NewVal"=w451:bool)  [unwired: 1 in]
        n277 = Unbundle("Motor") -> ("Value"=w450:dbl)  [unwired: 1 out]
        n278 = Select(t=w450, s=w451, f=0.0) -> (s? t:f=w448:dbl)
        n279 = call <vilib>:"NT Write Number.vi"("Numeric"=w448, "Name"=w447) -> ()  [unwired: 9 in, 1 out]
      }
      event "Test Slider": Value Change {
        # "When the test mode slider helper is set, update that\ntree row item's value"
        n280 = event-data() -> ("NewVal"=w455:dbl)  [unwired: 1 in]
        n281 = call <vilib>:"NT Write Number.vi"("Numeric"=w455, "Name"=w456) -> ()  [unwired: 9 in, 1 out]
      }
      event "On/Off": Value Change {
        # "When the test mode on/off helper value is set, update that\ntree row item's value"
        n282 = event-data() -> ("NewVal"=w461:bool)  [unwired: 1 in]
        n283 = Boolean To (0,1)(Boolean=w461) -> (0, 1=w460:i16)
        n284 = call <vilib>:"NT Write Number.vi"("Numeric"=w460, "Name"=w459) -> ()  [unwired: 9 in, 1 out]
      }
      event "Rev/Fwd": Value Change {
        # "When the test mode helper value for relays is set, update that\ntree row item's value"
        n285 = event-data() -> ("NewVal.Forward"=w470:bool, "NewVal.Reverse"=w469:bool)  [unwired: 1 in]
        n286 = Boolean To (0,1)(Boolean=w470) -> (0, 1=w466:i16)
        n287 = Boolean To (0,1)(Boolean=w469) -> (0, 1=w468:i16)
        n288 = Negate(x=w468) -> (-x=w467:i16)
        n289 = Add(x=w466, y=w467) -> (x+y=w465:i16)
        n290 = call <vilib>:"NT Write Number.vi"("Numeric"=w465, "Name"=w464) -> ()  [unwired: 9 in, 1 out]
      }
      event "Test Ring": Value Change {
        # "When a test mode helper value is selected from the ring,\nset the tree item's variable to the string value"
        n291 = event-data() -> ("NewVal"=w475:u16)  [unwired: 1 in]
        n292 = property on="Test Ring" class="Ring (strict)"() -> ("Strings []"=w476:string[])  [unwired: 2 in, 2 out]
        n293 = Index Array(array=w476, index=w475) -> (element=w474:string)
        n294 = call <vilib>:"NT Write String.vi"("String"=w474, "Name"=w473) -> ()  [unwired: 9 in, 1 out]
      }
      event "Rec Mode": Value Change {
        # "Update globals for recording mode and path to read log from.\nClear when logging and let NetworkTables set path for vision to\nuse."
        n295 = event-data() -> ("NewVal"=w488:enum32{"Stop", "Record", "Playback"})  [unwired: 1 in]
        n296 = global write "WPI_DashboardLogging Global.vi" "Logging Filename"(path "") -> ()
        n297 = global write "WPI_DashboardLogging Global.vi" "Recording"(w488) -> ()
        n298 = case shown="\"Playback\"" w488 {
          tunnel: w487 -> [_ w490 w499]
          tunnel: [_ _ w498] -> w484
          tunnel: [_ _ w497] -> _
          tunnel: w482 -> [_ _ w495]
          tunnel: cluster{i32, i32} {-250, 170} -> [_ _ w494]
          tunnel: [_ _ T23 {"Image Size"=TRUE, "Image Type"=TRUE, "Pixel Value"=TRUE, "ROI Information"=TRUE, "Zoom Factor"=FALSE} ("Image Information Shown:All Elements")] -> w480
          tunnel: [_ _ TRUE ("Zoom Factor")] -> w479
          tunnel: w478 -> [_ _ w491]
          frame Default {
          }
          frame "Stop", "Record" {
            # "Place Window too"
            n299 = invoke class="VI" method="FP.Close"(reference=w490) -> (reference out=w489:refnum<vi>)  [unwired: 2 in, 2 out]
            n300 = invoke class="VI" method="Abort VI"(reference=w489) -> ()  [unwired: 2 in, 3 out]
          }
          frame "Playback" {
            n301 = call "Open Playback Panel.vi"("Offset"=w494, "DB VI Ref"=w495, "Playback in"=w499) -> ("Playback out"=w496:refnum<vi>)  [unwired: 8 in]
            n302 = register-events(w496, w491) -> (reference out=w498:refnum<event-registration>, error out=w497:errorcluster)  [unwired: 2 in]
          }
        }
        n303 = property on="Camera Image" class="ImageControl"("Image Information Shown"=w480, "Image Information Visible"=w479) -> ()  [unwired: 2 in, 2 out]
        n304 = call <vilib>:"WPI_DashboardNT Log FieldName Cache.vi"("Operation"=enum16{"Lookup/Add", "Index", "Clear"}."Clear") -> ()  [unwired: 8 in, 3 out]
      }
      event Panel Close {
        w501 = enum32{"Stop", "Record", "Playback"}."Stop" ("Rec Mode")
        # "Playback window has been closed, abort"
        n305 = event-data() -> ()  [unwired: 1 in, 4 out]
        n306 = local write "Rec Mode"(w501) -> ()
        n307 = global write "WPI_DashboardLogging Global.vi" "Recording"(w501) -> ()
      }
      event Panel Close {
        # "Abort playback window and ourself"
        n308 = event-data() -> ()  [unwired: 1 in, 4 out]
        n309 = invoke class="VI" method="FP.Close"(reference=w507) -> (reference out=w506:refnum<vi>)  [unwired: 2 in, 2 out]
        n310 = invoke class="VI" method="Abort VI"(reference=w506) -> (error out=w505:errorcluster)  [unwired: 2 in, 2 out]
        n311 = invoke class="VI" method="Abort VI"(error in=w505) -> ()  [unwired: 2 in, 3 out]
      }
      event User Event {
        n312 = event-data() -> ("IDs"=w515:cluster{"RPC field ID":u16, "Unique ID":u16}, "String"=w514:string)  [unwired: 1 in]
        n313 = Bundle("IDs"=w515, "String"=w514) -> (w513:T9)  [unwired: 1 in]
        n314 = call <vilib>:"Retrieve RPC Response.vi"("RPC Response"=w513) -> ("Output"=w510:string[][])  [unwired: 10 in]
        n315 = Build Array (concatenate)(w508, w510) -> (w509:string[][])
        n316 = local write "Command Params"(w509) -> ()
        n317 = local write "Cmd Status"("" ("Cmd Status")) -> ()
      }
      event "Vision": Value Change {
        # "Enable/Disable Compression slider.\nHW USB is hard-coded into the camera"
        n318 = event-data() -> ("NewVal"=w522:u16)  [unwired: 1 in]
        n319 = Equal?(x=w522, y=u32 2 ("milliseconds to wait")) -> (x = y?=w520:bool)
        n320 = Select(t=T24."Disabled and Grayed Out" ("Disabled"), s=w520, f=T24."Enabled" ("Disabled")) -> (s? t:f=w517:T24)
        n321 = property on="Compression" class="Slide (strict)"("DisabledEnum"=w517) -> ()  [unwired: 2 in, 2 out]
      }
      event "Tree": Double Click {
        n322 = event-data() -> ("PlatMods"=w527:T27, "Tag"=w526:string)  [unwired: 1 in]
        n323 = Unbundle(w527) -> ("Shift"=w525:bool)  [unwired: 4 out]
        n324 = Not(x=w525) -> (.not. x?=w524:bool)
        n325 = call <vilib>:"NT Update Persistence.vi"("Persistence"=w524, "Name"=w526) -> ()  [unwired: 9 in, 1 out]
      }
    }
  }
  n326 = while {
    tunnel: w47 -> [w531]
    i -> [w534]
    stop <- FALSE stop-if-true
    n327 = Wait (ms)(milliseconds to wait=u32 100) -> ()  [unwired: 1 out]
    n328 = case shown="\"Stop\", Default" "Rec Mode" {
      tunnel: w534 -> [_ _ w547]
      tunnel: [u32 2829099 ("Base Color") u32 11141120 ("Target Color") w538] -> w530
      frame "Stop", Default {
        # "Reset the color, extra updates don't cost much"
      }
      frame "Record" {
      }
      frame "Playback" {
        # "Playback"
        n329 = Quotient & Remainder(x=w547, y=u32 50 ("milliseconds to wait")) -> (x-y*floor(x/y)=w544:u32)  [unwired: 1 out]
        n330 = Divide(x=w544, y=u32 50 ("milliseconds to wait")) -> (x/y=w541:dbl)
        n331 = Multiply(x=6.283185307179586, y=w541) -> (x*y=w545:dbl)
        n332 = Sine(x=w545) -> ()  [unwired: 1 out]
        n333 = call "Interpolate RGB Color.vi"("Target Color"=u32 30976, "Base Color"=u32 2829099) -> ("Result Color"=w538:u32)  [unwired: 9 in]
      }
    }
    n334 = property class="Pane"(reference=w531, "PaneColor"=w530) -> ()  [unwired: 1 in, 2 out]
  }
  n335 = local write "Dashboard Tab"(T2."Drive" ("Dashboard Tab")) -> ()
  n336 = property on="On/Off" class="Bool (strict)"("Visible"=w15) -> ()  [unwired: 2 in, 2 out]
  n337 = property on="Motor" class="Clust (strict)"("Visible"=w15) -> ()  [unwired: 2 in, 2 out]
  n338 = property on="Progress" class="Clust (strict)"("Visible"=w15) -> ()  [unwired: 2 in, 2 out]
  n339 = property on="Test Ring" class="Ring (strict)"("Visible"=w15) -> ()  [unwired: 2 in, 2 out]
  n340 = property on="Rev/Fwd" class="Clust (strict)"("Visible"=w15) -> ()  [unwired: 2 in, 2 out]
  n341 = property on="Camera Settings" class="Clust (strict)"("Visible"=w15) -> ()  [unwired: 2 in, 2 out]
  n342 = local write "DB Camera Config"(w15) -> ()
  n343 = local write "Command Params"(string[][] [] ("Command Params")) -> ()
  n344 = global write "WPI_DashboardLogging Global.vi" "Recording"(w41) -> ()
  n345 = local write "Rec Mode"(w41) -> ()
  n346 = while {
    tunnel: u16 1741 ("timeout ms (25000)") -> [w549]
    stop <- FALSE stop-if-true
    n347 = TCP Create Listener(10:w549) -> (0:w548:errorcluster, 3:w550:refnum<k5>)  [unwired: 4 in, 1 out]
    n348 = case shown="No Error" w548 {
      selector: w548 -> [w552 _]
      tunnel: w550 -> [w553 _]
      frame No Error {
        n349 = while {
          tunnel: w553 -> [w556]
          tunnel: w552 -> [w555]
          stop <- FALSE stop-if-true
          n350 = TCP Wait On Listener(8:w555, 11:w556) -> (0:w557:errorcluster, 4:w558:refnum<k5>)  [unwired: 2 in, 3 out]
          n351 = local write "TCP"(w558) -> ()
          n352 = case shown="No Error" w557 {
            frame No Error {
            }
            frame Error {
              n353 = Wait (ms)(milliseconds to wait=u32 1000) -> ()  [unwired: 1 out]
            }
          }
        }
      }
      frame Error {
        n354 = Wait (ms)(milliseconds to wait=u32 1000) -> ()  [unwired: 1 out]
      }
    }
  }
  n355 = local write "Command Selection"(u16 0 ("milliseconds to wait")) -> ()
  n356 = while {
    tunnel: [w569] -> _
    i -> [w569]
    stop <- FALSE stop-if-true
    # "Optionally read the DB image,\nlog, or retrieve images from a\nlogged match"
    n357 = local read "Rec Mode"() -> (w564:enum32{"Stop", "Record", "Playback"})
    n358 = local read "Camera IP"() -> (w562:string)
    n359 = call <vilib>:"WPI_CameraRead MJPG for Dashboard.vi"("Camera Settings"="Camera Settings 2", "Rec Mode"=w564, "Camera IP"=w562, "Camera Mode"="Vision 2") -> ("Active"=w567:bool, "Refnum out"=w568:T1, "FPS"=w566:dbl, "Bandwidth (Mbps)"=w561:dbl)  [unwired: 4 in]
    "Mbps 2" <- w561
    n360 = case shown="True" w567 {
      tunnel: w568 -> [_ w578]
      tunnel: w561 -> [_ w577]
      tunnel: w566 -> [_ w576]
      frame False {
        w571 = u32 1985280 ("Color Box")
        # "Sleep for 500ms"
        n361 = Bundle("Color Box"=w571, "Color Box"=w571) -> (w573:cluster{"Color Box":u32, "Color Box":u32})  [unwired: 1 out]
        n362 = Build Array(w573) -> (w572:cluster{"Color Box":u32, "Color Box":u32}[])
        n363 = property on="Mbps LED" class="Bool (strict)"("Colors [4]"=w572) -> ()  [unwired: 2 in, 2 out]
        n364 = Wait Until Next ms Multiple(millisecond multiple=u32 500) -> ()  [unwired: 1 out]
      }
      frame True {
        # "Here is where you would annotate,\npossibly process, and display the image"
        # "Update Mbps LED"
        n365 = call "IMAQ Clear Overlay"("Image"=w578) -> ("error out"=w582:errorcluster, "Image Out"=→"Camera Image 2":T1)  [unwired: 2 in, 7 out]
        n366 = case shown="Default" w577 {
          tunnel: [u32 6618880 ("Color Box") u32 16776722 ("Color Box") u32 16716800 ("Color Box")] -> w579
          frame Default {
          }
          frame 4, 5 {
          }
          frame 6.. {
          }
        }
        n367 = Unbundle By Name(w582) -> ("status"=w583:bool)
        n368 = Bundle("Color Box"=w579, "Color Box"=w579) -> (w581:cluster{"Color Box":u32, "Color Box":u32})  [unwired: 1 out]
        n369 = property on="Image Message" class="Str"("Visible"=w583) -> ()  [unwired: 2 in, 2 out]
        n370 = Build Array(w581) -> (w580:cluster{"Color Box":u32, "Color Box":u32}[])
        n371 = property on="Mbps LED" class="Bool (strict)"("Colors [4]"=w580) -> ()  [unwired: 2 in, 2 out]
        "fps 2" <- w576
      }
    }
  }
